vi "Volume Matcher.vi"() -> ()   [LabVIEW 2024, in "CLZ_to_ComicVine.lvlib"]
uses:
  CLZ_to_ComicVine.lvlib
  Volumes/CV Comics.lvclass
  CLZ Comics/CLZ Comics.lvclass
  <vilib>/Utility/miscctls.llb/LVRowAndColumnUnsignedTypeDef.ctl
  <vilib>/addons/_JKI Toolkits/State Machine/_JKI_lib_State_Machine.llb/Select State(s)_err__jki_lib_state_machine.vi
  <vilib>/addons/_JKI Toolkits/State Machine/_JKI_lib_State_Machine.llb/Periodic Trigger__ogtk__JKI-SM__jki_lib_state_machine.vi
panel:
  in  "Matched Volumes":i32(listbox)
  in  "CLZ Issues":i32(listbox)
  in  "regex":string
  in  "Sort Type":enum16{"Fuzzy", "Regex"}(ring)
  in  "refresh":bool
  in  "compare threshold":dbl=0.5 min=0.0 max=1.0 step=0.1
  out "progress":i32(slide) caption="1582 of 1626" scale=0.0..1626.0
  in  "Remove Set":bool
  in  "Apply Set":bool
  in  "CV Volumes":i32(listbox)
  in  "CLZ Volumes":i32(listbox)
  in  "Exit":bool
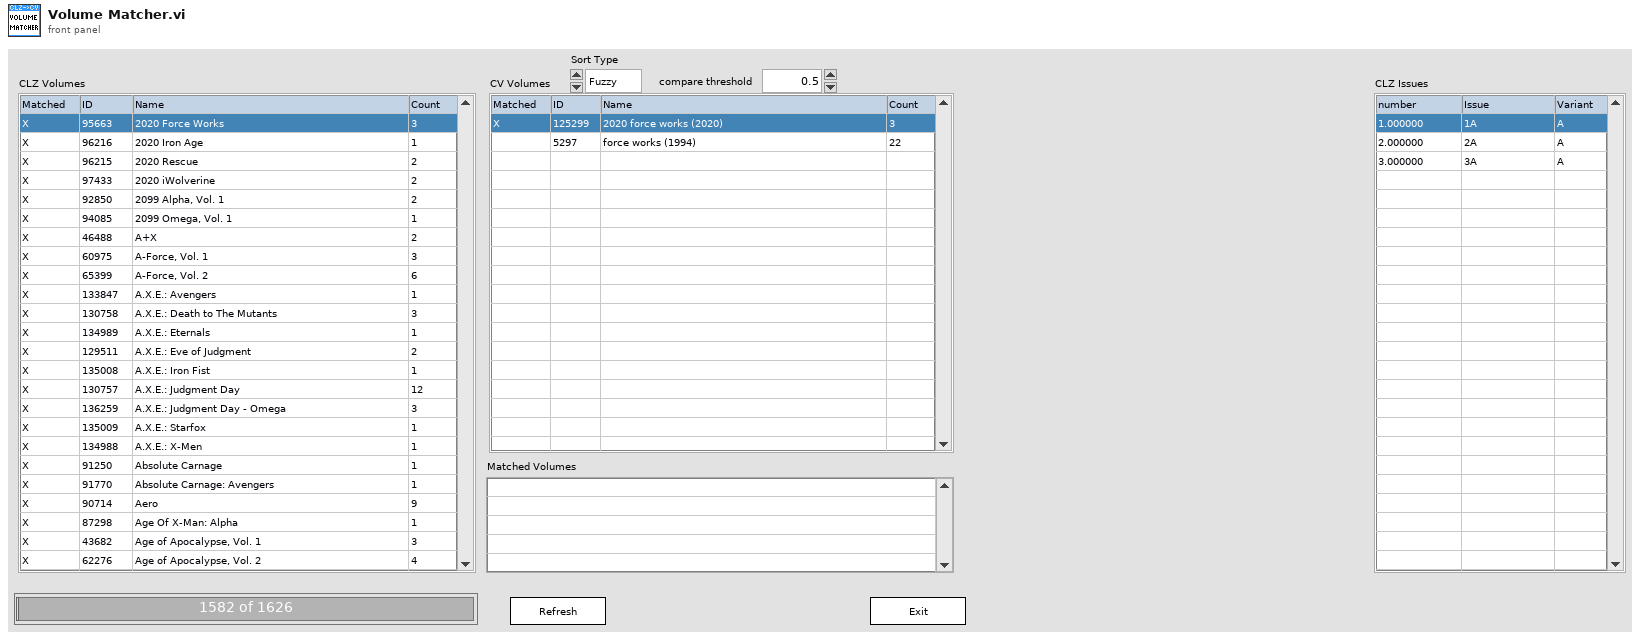
[diagram p1: front panel]
types:
  T1 = enum32{"Invalid", "Standard", "Closed", "Hidden", "Minimized", "Maximized"}
  T2 = enum32{"invalid app kind", "Development System", "Run Time System", "Student Edition", "Embedded LabVIEW", "Evaluation", "Custom"}
  T3 = cluster{"Core":cluster{"Current VI Reference":refnum<vi>, "Close Panel on Exit?":bool}, "CLZ report path":path, "CV binary folder":path, "matched set":set{cluster{"CLZ ID":i32, "CV ID":i32}}, "CLZ Comics":refnum<class "CLZ Comics.lvclass">, "CV volumes":refnum<class "CV Comics.lvclass">}
  T4 = cluster{"Current VI Reference":refnum<vi>, "Close Panel on Exit?":bool}
  T5 = typedef "LVRowAndColumnUnsignedTypeDef.ctl" = cluster{"Row":u32, "Column":u32}
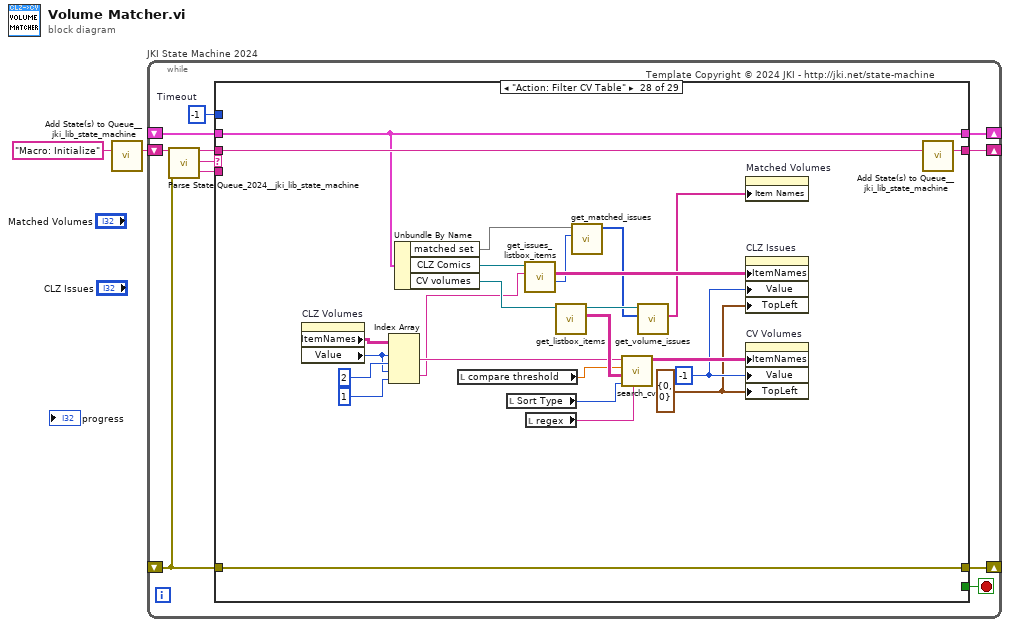
[diagram p0: block diagram]
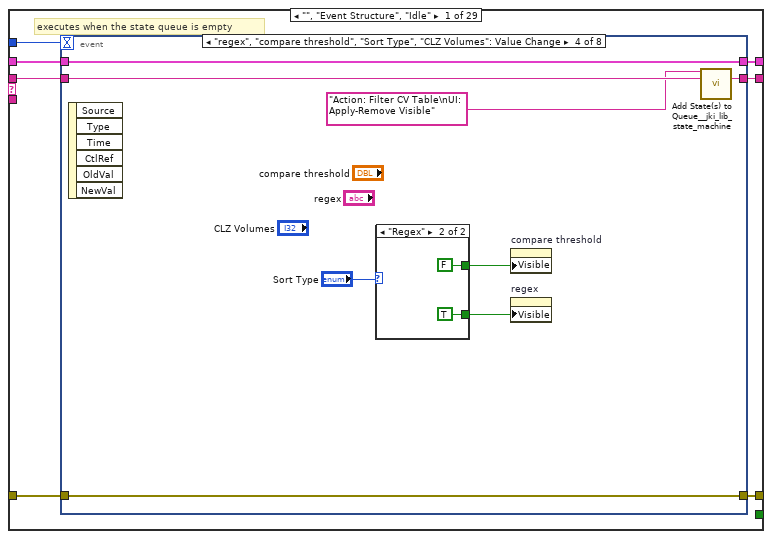
[diagram p2: hidden frame]
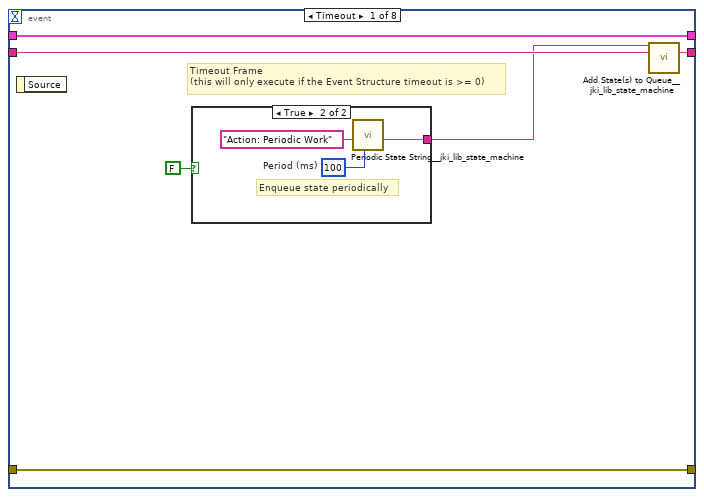
[diagram p3: hidden frame]
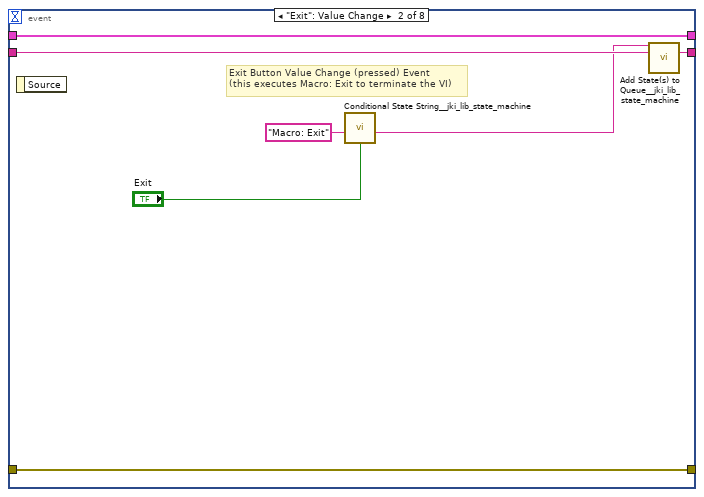
[diagram p5: hidden frame]
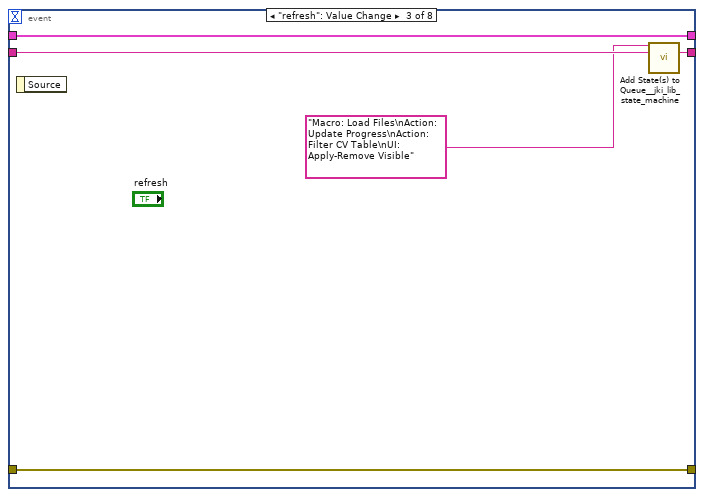
[diagram p6: hidden frame]
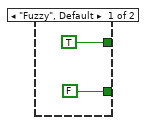
[diagram p7: hidden frame]
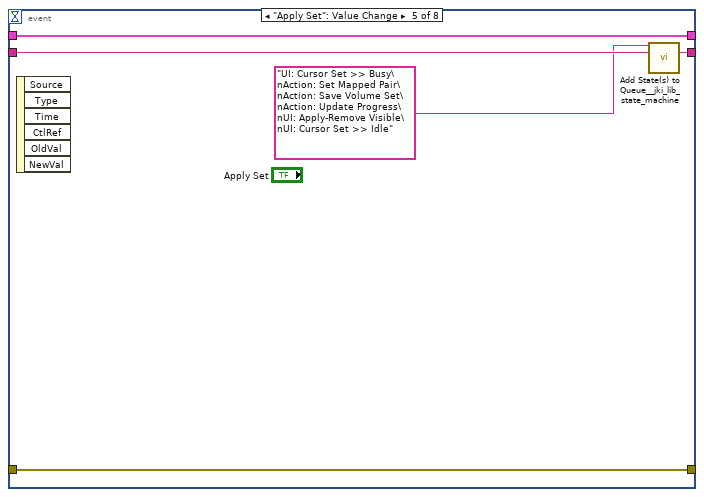
[diagram p8: hidden frame]
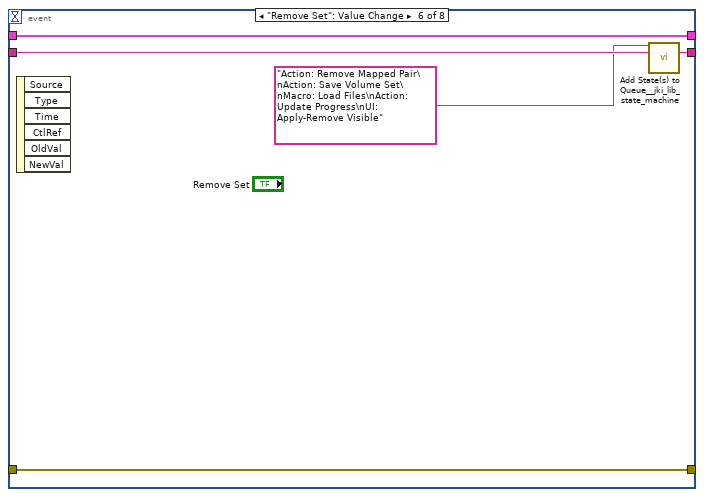
[diagram p9: hidden frame]
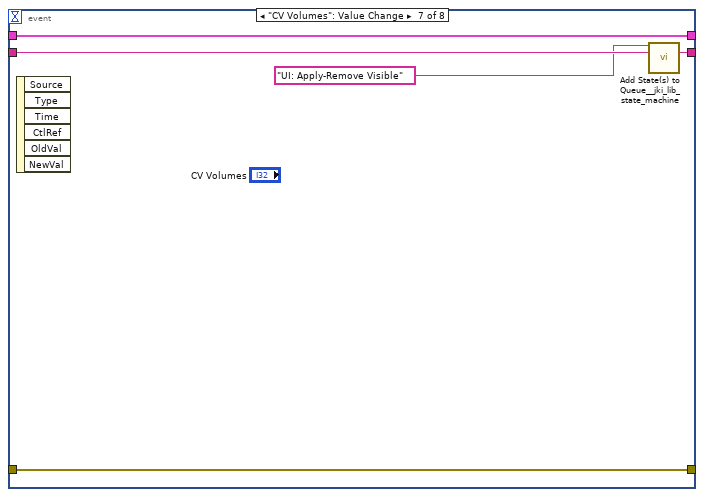
[diagram p10: hidden frame]
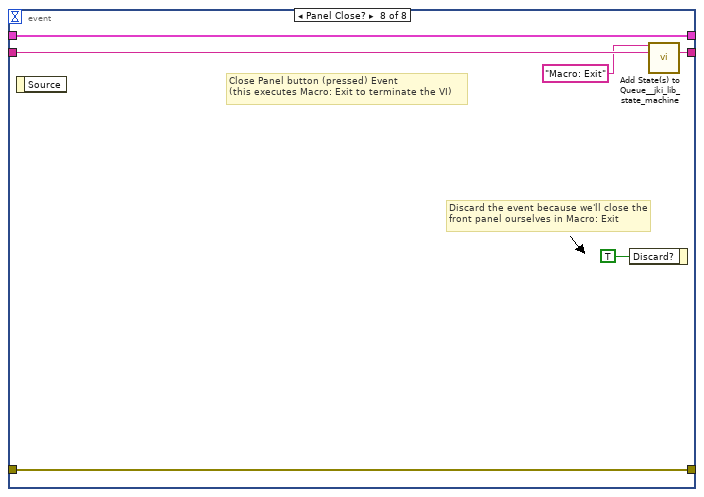
[diagram p11: hidden frame]
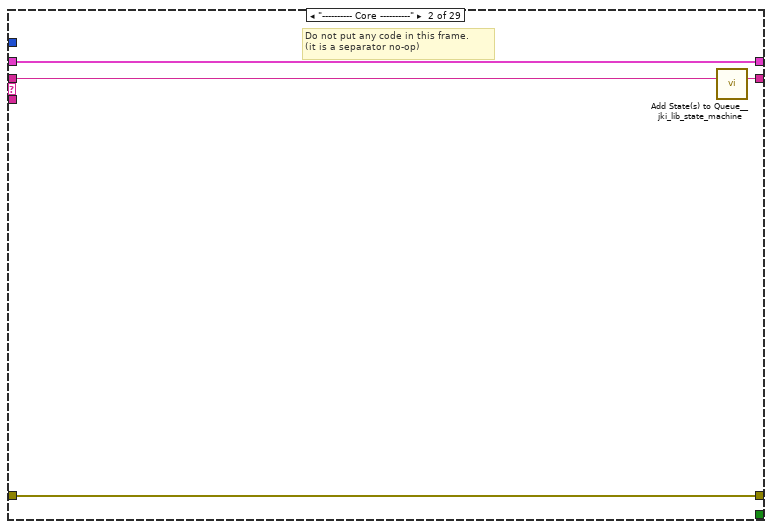
[diagram p12: hidden frame]
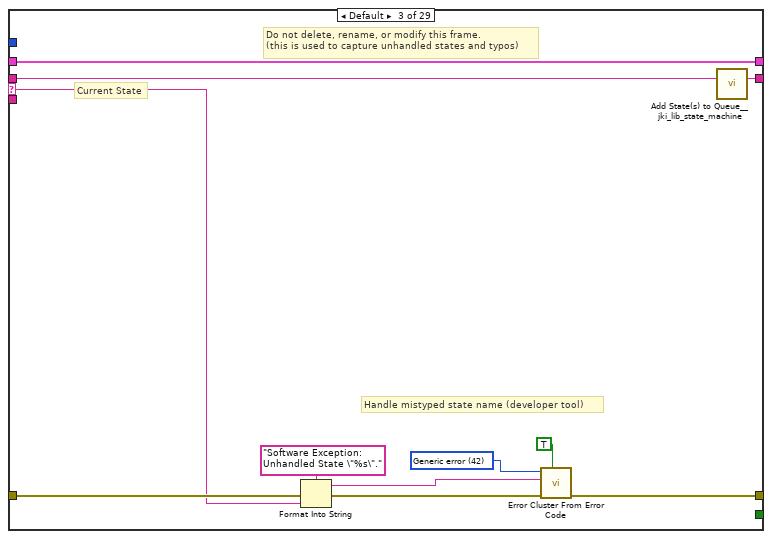
[diagram p13: hidden frame]
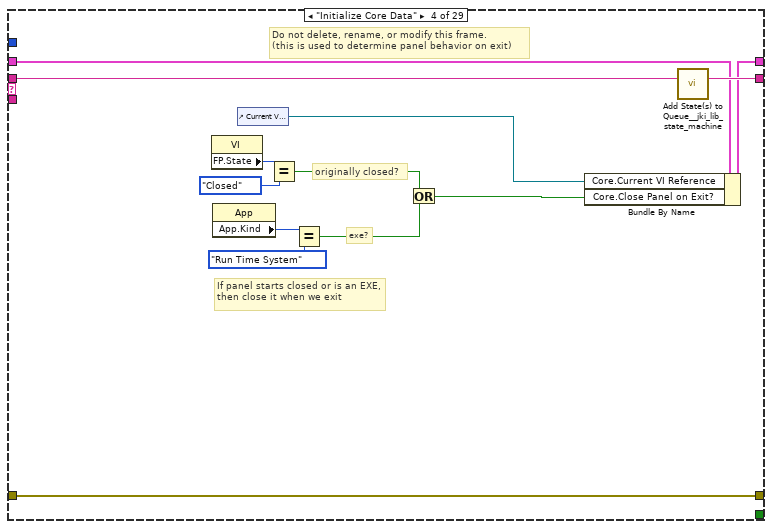
[diagram p14: hidden frame]
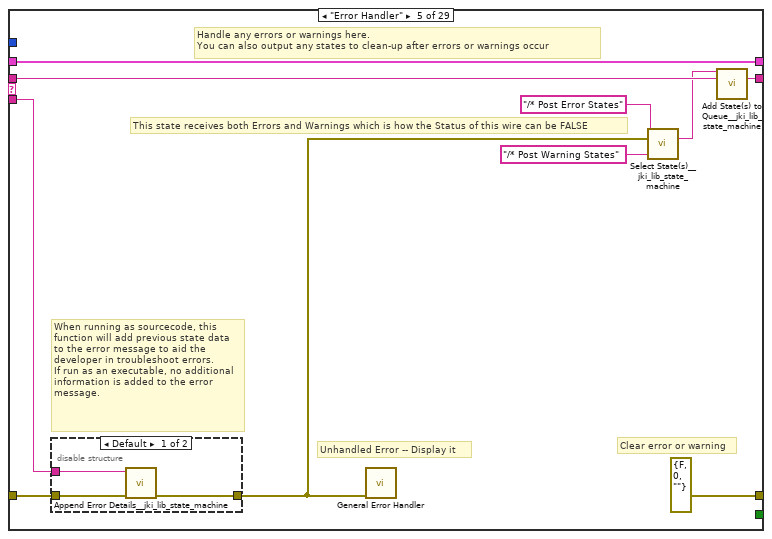
[diagram p15: hidden frame]
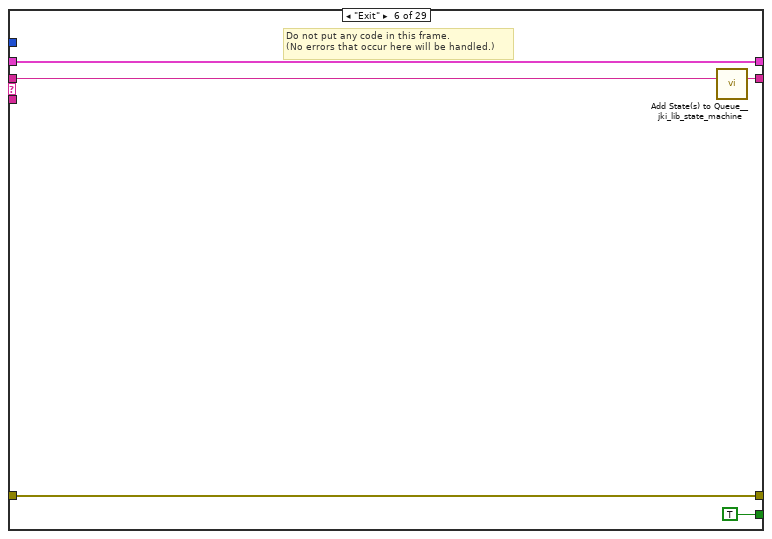
[diagram p17: hidden frame]
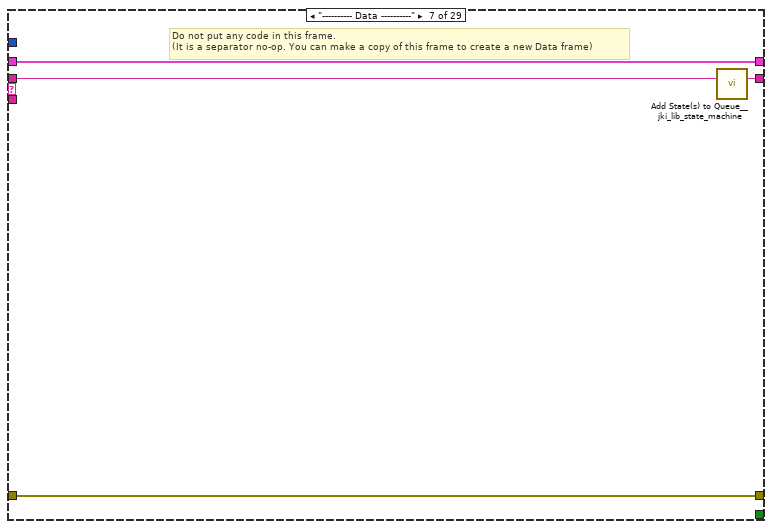
[diagram p18: hidden frame]
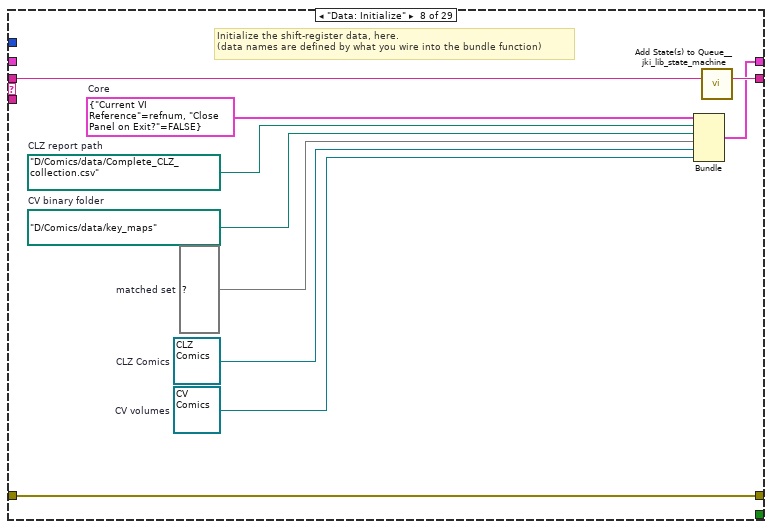
[diagram p19: hidden frame]
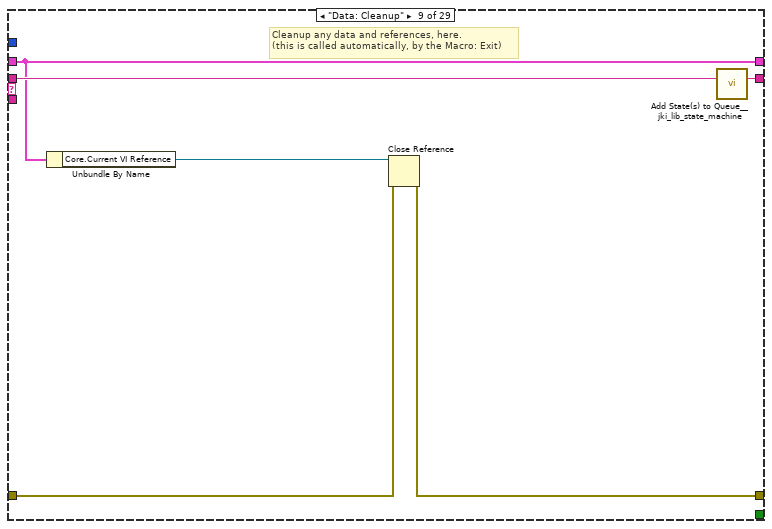
[diagram p20: hidden frame]
diagram:
  n1 = call <vilib>:"Add State(s) to Queue__jki_lib_state_machine.vi"("State(s) in (\"\")"="Macro: Initialize") -> ("States Out"=w2:string)  [unwired: 14 in]
  n2 = while "JKI State Machine 2024" {
    shift-right: [w6] -> _
    shift-left: _ -> [w5]
    shift-right: [w9] -> _
    shift-left: _ -> [w3]
    shift-right: [w8] -> _
    shift-left: w2 -> [w10]
    stop <- w7 stop-if-true
    w4 = -1  # Timeout
    # "Template Copyright © 2024 JKI - http://jki.net/state-machine"
    n3 = call <vilib>:"Parse State Queue_2024__jki_lib_state_machine.vi"("State Queue"=w10, "Error In (no error)"=w3) -> ("Remaining States"=w12:string, "Current State"=w13:string, "Arguments"=w11:string)  [unwired: 11 in]
    n4 = case shown="\"Action: Filter CV Table\"" w13 {
      selector: w13 -> [_ _ w79 _ _ _ _ _ _ _ _ _ _ _ _ _ _ _ _ _ _ _ _ _ _ _ _ _ _]
      tunnel: w12 -> [w20 w78 w83 w102 w112 w121 w125 w135 w141 w145 w167 w195 w201 w207 w218 w287 w292 w297 w306 w310 w317 w343 w365 w376 w386 w394 w403 w428 w438]
      tunnel: w11 -> [_ _ _ _ w107 _ _ _ _ _ _ _ _ w202 w212 _ _ _ _ _ _ _ _ _ _ _ _ _ _]
      tunnel: w5 -> [w18 w75 w81 w95 w109 w119 w122 _ w136 w142 w158 w193 w199 w205 w214 w284 w289 w294 w304 w307 w315 w327 w362 w374 w384 w392 w401 w423 w436]
      tunnel: [w17 w76 w85 w99 errorcluster {"status"=FALSE, "code"=0, "source"=""} ("error out") w118 w123 w132 w137 w143 w165 w192 w198 w203 w215 w285 w290 w295 w301 w308 w311 w341 w363 w370 w377 w387 w397 w426 w433] -> w9
      tunnel: w3 -> [w14 w76 w84 w99 w108 w118 w123 w132 w138 w143 w165 w192 w198 w204 w216 w285 w290 w295 w301 w308 w312 w341 w363 w373 w378 w388 w398 w426 w435]
      tunnel: [w19 w77 w82 w101 w111 w120 w124 w134 w140 w144 w166 w194 w200 w206 w217 w286 w291 w296 w305 w309 w316 w342 w364 w375 w385 w393 w402 w427 w437] -> w8
      tunnel: [_ _ _ _ _ TRUE _ _ _ _ _ _ _ _ _ _ _ _ _ _ _ _ _ _ _ _ _ _ _] -> w7
      tunnel: [w16 w75 w81 w100 w109 w119 w122 w133 w136 w142 w158 w193 w199 w205 w214 w284 w289 w294 w304 w307 w315 w326 w361 w374 w383 w391 w401 w423 w434] -> w6
      tunnel: w4 -> [w15 _ _ _ _ _ _ _ _ _ _ _ _ _ _ _ _ _ _ _ _ _ _ _ _ _ _ _ _]
      frame "", "Event Structure", "Idle" {
        # "executes when the state queue is empty"
        n5 = event shown="[3] \"regex\", \"compare threshold\", \"Sort Type\", \"CLZ Volumes\": Value Change" {
          selector: _ -> [_ _ _ _ _ _ _ _]
          dyn-events: _ -> [_ _ _ _ _ _ _ _]
          timeout: w15 -> [_ _ _ _ _ _ _ _]
          tunnel: w20 -> [w26 w36 w41 w49 w58 w63 w68 w74]
          tunnel: [w25 w35 w40 w48 w57 w62 w67 w73] -> w19
          tunnel: w18 -> [w23 w33 w38 w46 w55 w60 w65 w71]
          tunnel: [w24 w34 w39 w47 w56 w61 w66 w72] -> w17
          tunnel: w14 -> [w24 w34 w39 w47 w56 w61 w66 w72]
          tunnel: [w23 w33 w38 w46 w55 w60 w65 w71] -> w16
          event Timeout {
            # "Timeout Frame\n(this will only execute if the Event Structure timeout is >= 0)"
            n6 = event-data() -> ()  [unwired: 1 in, 1 out]
            n7 = case shown="True" FALSE {
              tunnel: [_ w29] -> w22
              frame False {
              }
              frame True {
                w27 = u32 100  # Period (ms)
                # "Enqueue state periodically"
                n8 = call <vilib>:"Periodic State String__jki_lib_state_machine.vi"("Period (ms)"=w27, "State"="Action: Periodic Work") -> ("State Out"=w29:string)  [unwired: 9 in]
              }
            }
            n9 = call <vilib>:"Add State(s) to Queue__jki_lib_state_machine.vi"("State(s) in Front (\"\")"=w22, "State(s) in (\"\")"=w26) -> ("States Out"=w25:string)  [unwired: 13 in]
          }
          event "Exit": Value Change {
            # "Exit Button Value Change (pressed) Event\n(this executes Macro: Exit to terminate the VI)"
            n10 = event-data() -> ()  [unwired: 1 in, 1 out]
            n11 = call <vilib>:"Conditional State String__jki_lib_state_machine.vi"("Do State(s)?"="Exit", "State"="Macro: Exit") -> ("State Out"=w30:string)  [unwired: 7 in]
            n12 = call <vilib>:"Add State(s) to Queue__jki_lib_state_machine.vi"("State(s) in Front (\"\")"=w30, "State(s) in (\"\")"=w36) -> ("States Out"=w35:string)  [unwired: 13 in]
          }
          event "refresh": Value Change {
            n13 = event-data() -> ()  [unwired: 1 in, 1 out]
            n14 = call <vilib>:"Add State(s) to Queue__jki_lib_state_machine.vi"("State(s) in Front (\"\")"="Macro: Load Files\nAction: Update Progress\nAction: Filter CV Table\nUI: Apply-Remove Visible" ("State(s) in Front (\"\")"), "State(s) in (\"\")"=w41) -> ("States Out"=w40:string)  [unwired: 13 in]
          }
          event "regex", "compare threshold", "Sort Type", "CLZ Volumes": Value Change {
            n15 = event-data() -> ()  [unwired: 1 in, 6 out]
            n16 = case shown="\"Regex\"" "Sort Type" {
              tunnel: [TRUE FALSE] -> w44
              tunnel: [FALSE TRUE] -> w43
              frame "Fuzzy", Default {
              }
              frame "Regex" {
              }
            }
            n17 = property on="compare threshold" class="DigNum (strict)"("Visible"=w44) -> ()  [unwired: 2 in, 2 out]
            n18 = property on="regex" class="Str"("Visible"=w43) -> ()  [unwired: 2 in, 2 out]
            n19 = call <vilib>:"Add State(s) to Queue__jki_lib_state_machine.vi"("State(s) in Front (\"\")"="Action: Filter CV Table\nUI: Apply-Remove Visible", "State(s) in (\"\")"=w49) -> ("States Out"=w48:string)  [unwired: 13 in]
          }
          event "Apply Set": Value Change {
            n20 = event-data() -> ()  [unwired: 1 in, 6 out]
            n21 = call <vilib>:"Add State(s) to Queue__jki_lib_state_machine.vi"("State(s) in Front (\"\")"="UI: Cursor Set >> Busy\nAction: Set Mapped Pair\nAction: Save Volume Set\nAction: Update Progress\nUI: Apply-Remove Visible\nUI: Cursor Set >> Idle", "State(s) in (\"\")"=w58) -> ("States Out"=w57:string)  [unwired: 13 in]
          }
          event "Remove Set": Value Change {
            n22 = event-data() -> ()  [unwired: 1 in, 6 out]
            n23 = call <vilib>:"Add State(s) to Queue__jki_lib_state_machine.vi"("State(s) in Front (\"\")"="Action: Remove Mapped Pair\nAction: Save Volume Set\nMacro: Load Files\nAction: Update Progress\nUI: Apply-Remove Visible", "State(s) in (\"\")"=w63) -> ("States Out"=w62:string)  [unwired: 13 in]
          }
          event "CV Volumes": Value Change {
            n24 = event-data() -> ()  [unwired: 1 in, 6 out]
            n25 = call <vilib>:"Add State(s) to Queue__jki_lib_state_machine.vi"("State(s) in Front (\"\")"="UI: Apply-Remove Visible", "State(s) in (\"\")"=w68) -> ("States Out"=w67:string)  [unwired: 13 in]
          }
          event Panel Close? {
            # "Discard the event because we'll close the front panel ourselves in Macro: Exit"
            # "Close Panel button (pressed) Event\n(this executes Macro: Exit to terminate the VI)"
            n26 = event-data() -> ()  [unwired: 1 in, 1 out]
            n27 = event-data("Discard?"=TRUE) -> ()  [unwired: 1 in, 1 out]
            n28 = call <vilib>:"Add State(s) to Queue__jki_lib_state_machine.vi"("State(s) in Front (\"\")"="Macro: Exit", "State(s) in (\"\")"=w74) -> ("States Out"=w73:string)  [unwired: 13 in]
          }
        }
      }
      frame "---------- Core ----------" {
        # "Do not put any code in this frame.\n(it is a separator no-op)"
        n29 = call <vilib>:"Add State(s) to Queue__jki_lib_state_machine.vi"("State(s) in (\"\")"=w78) -> ("States Out"=w77:string)  [unwired: 14 in]
      }
      frame Default {
        w88 = 42 items=["No error", "Argument error", "Memory is full", "Out of zone", "End of file", "File already open", "Generic file I/O error", "File not found", "File permission error", "Disk is full", "Duplicate path", "Too many files open", "System feature not enabled", "Resource file not found", "Cannot add resource", "Resource not found", "Image not found", "Image memory error", "Pen does not exist", "Config type invalid", "Config token not found", "Config parse error", "Config memory error", "Bad external code format", "Bad external code offset", "External code not present", "Null window", "Destroy window error", "Null menu", "Print aborted", "Bad print record", "Print driver error", "Windows error during printing", "Memory error during printing", "Print dialog error", "Generic print error", "Invalid device refnum", "Device not found", "Device parameter error", "Device unit error", "Cannot open device", "Device call aborted", "Generic error", "Cancelled by user", "Object ID too low", "Object ID too high", "Object not in heap", "Unknown heap", "Unknown object (invalid DefProc)", "Unknown object (DefProc not in table)", "Message out of range", "Invalid (null) method", "Unknown message", "Manager call not supported", "Bad address", "Network operation in progress", "Network operation timed out", "Connection is busy", "Network attribute not supported", "Network error", "Address in use", "System out of memory", "Connection aborted", "Connection refused", "Not connected", "Already connected", "Connection closed", "Initialization error (interapplication manager)", "Bad occurrence", "Wait on unbound occurrence handler", "Occurrence queue overflow", "Datalog type conflict", "Unused", "Unrecognized type (interapplication manager)", "Memory corrupt", "Failed to make temporary DLL", "Old CIN version", "Drag socket not found", "Failed to load drop-object", "Failed to register OLE object", "Failed to release OLE object", "Format specifier type mismatch", "Unknown format specifier", "Too few format specifiers", "Too many format specifiers", "Scan failed", "Newer CIN version", "Error converting to variant", "Runtime menu error", "Password tampered", "Variant attribute not found", "Incompatible variant data type", "Event data is not available", "Event Store is not present", "Occurrence is not found", "Event Queue is not created", "Event info is not available", "Refnum passed is NULL", "Error retrieving Class GUID", "Error retrieving CoClass GUID", "Error retrieving TypeLib GUID.", "Bad built application magic bytes.", "Specific driver is different from the specific driver associated with the Logical Name.", "There is no session opened to the class driver.", "Max Error", "MAX - Error with config objects", "MAX - Error loading configuration", "MAX - Group not supported"]
        # "Current State"
        # "Do not delete, rename, or modify this frame.\n(this is used to capture unhandled states and typos)"
        # "Handle mistyped state name (developer tool)"
        n30 = Format Into String(format string="Software Exception: Unhandled State \"%s\"." ("message"), error in=w84, w79) -> (resulting string=w87:string, error out=w86:errorcluster)  [unwired: 1 in]
        n31 = call <vilib>:"Error Cluster From Error Code.vi"("show call chain? (False)"=TRUE, "error in (no error)"=w86, "error message (\"\")"=w87, "error code (0)"=w88) -> ("error out"=w85:errorcluster)  [unwired: 5 in]
        n32 = call <vilib>:"Add State(s) to Queue__jki_lib_state_machine.vi"("State(s) in (\"\")"=w83) -> ("States Out"=w82:string)  [unwired: 14 in]
      }
      frame "Initialize Core Data" {
        # "Do not delete, rename, or modify this frame.\n(this is used to determine panel behavior on exit)"
        # "originally closed?"
        # "exe?"
        # "If panel starts closed or is an EXE, then close it when we exit"
        n33 = property class="VI"() -> ("FP.State"=w92:T1)  [unwired: 2 in, 2 out]
        n34 = property class="App"() -> ("App.Kind"=w98:T2)  [unwired: 2 in, 2 out]
        n35 = control-ref of="Current VI Reference"() -> (w93:refnum<vi>)
        n36 = Equal?(x=w92, y=T1."Closed" ("Front Panel Window:State")) -> (x = y?=w90:bool)
        n37 = Equal?(x=w98, y=T2."Run Time System" ("Application:Kind")) -> (x = y?=w96:bool)
        n38 = Or(x=w90, y=w96) -> (x .or. y?=w94:bool)
        n39 = Bundle By Name(cluster=w95, "Core.Current VI Reference"=w93, "Core.Close Panel on Exit?"=w94) -> (w100:T3)
        n40 = call <vilib>:"Add State(s) to Queue__jki_lib_state_machine.vi"("State(s) in (\"\")"=w102) -> ("States Out"=w101:string)  [unwired: 14 in]
      }
      frame "Error Handler" {
        # "When running as sourcecode, this function will add previous state data to the error message to aid the developer in troubleshoot errors.\nIf run as an executable, no additional information is added to the error message."
        # "This state receives both Errors and Warnings which is how the Status of this wire can be FALSE"
        # "Unhandled Error -- Display it"
        # "Handle any errors or warnings here.\nYou can also output any states to clean-up after errors or warnings occur"
        # "Clear error or warning"
        n41 = disable-structure shown="Default" {
          disable-tunnel: w108 -> [w115 w116]
          disable-tunnel: w107 -> [w114 _]
          disable-tunnel: [w113 w116] -> w106
          frame condition #0 (active) {
            n42 = call <vilib>:"Append Error Details__jki_lib_state_machine.vi"("error in (no error)"=w115, "Previous State and Argument(s)"=w114) -> ("error out"=w113:errorcluster)  [unwired: 9 in]
          }
          frame condition #1 {
          }
        }
        n43 = call <vilib>:"General Error Handler.vi"("error in (no error)"=w106) -> ()  [unwired: 10 in, 5 out]
        n44 = call-poly <vilib>:"Select State(s)__jki_lib_state_machine.vi"("State(s) if True (\"\")"="/* Post Error States", "Select"=w106, "State(s) if False (\"\")"="/* Post Warning States") -> ("States Out"=w104:string)  [unwired: 12 in]
        n45 = call <vilib>:"Add State(s) to Queue__jki_lib_state_machine.vi"("State(s) in Front (\"\")"=w104, "State(s) in (\"\")"=w112) -> ("States Out"=w111:string)  [unwired: 13 in]
      }
      frame "Exit" {
        # "Do not put any code in this frame.\n(No errors that occur here will be handled.)"
        n46 = call <vilib>:"Add State(s) to Queue__jki_lib_state_machine.vi"("State(s) in (\"\")"=w121) -> ("States Out"=w120:string)  [unwired: 14 in]
      }
      frame "---------- Data ----------" {
        # "Do not put any code in this frame.\n(It is a separator no-op. You can make a copy of this frame to create a new Data frame)"
        n47 = call <vilib>:"Add State(s) to Queue__jki_lib_state_machine.vi"("State(s) in (\"\")"=w125) -> ("States Out"=w124:string)  [unwired: 14 in]
      }
      frame "Data: Initialize" {
        w126 = refnum<class "CLZ Comics.lvclass"> refnum  # CLZ Comics
        w127 = refnum<class "CV Comics.lvclass"> refnum  # CV volumes
        w128 = set{cluster{"CLZ ID":i32, "CV ID":i32}} {}  # matched set
        w129 = path "D:/Comics/data/key_maps"  # CV binary folder
        w130 = path "D:/Comics/data/Complete_CLZ_collection.csv"  # CLZ report path
        w131 = T4 {"Current VI Reference"=refnum, "Close Panel on Exit?"=FALSE}  # Core
        # "Initialize the shift-register data, here.\n(data names are defined by what you wire into the bundle function)"
        n48 = Bundle("Core"=w131, "CLZ report path"=w130, "CV binary folder"=w129, "matched set"=w128, "CLZ Comics"=w126, "CV volumes"=w127) -> (w133:T3)  [unwired: 1 in]
        n49 = call <vilib>:"Add State(s) to Queue__jki_lib_state_machine.vi"("State(s) in (\"\")"=w135) -> ("States Out"=w134:string)  [unwired: 14 in]
      }
      frame "Data: Cleanup" {
        # "Cleanup any data and references, here.\n(this is called automatically, by the Macro: Exit)"
        n50 = Unbundle By Name(w136) -> ("Core.Current VI Reference"=w139:refnum<vi>)
        n51 = Close Reference(reference=w139, error in (no error)=w138) -> (error out=w137:errorcluster)
        n52 = call <vilib>:"Add State(s) to Queue__jki_lib_state_machine.vi"("State(s) in (\"\")"=w141) -> ("States Out"=w140:string)  [unwired: 14 in]
      }
      frame "---------- UI ----------" {
        # "Do not put any code in this frame.\n(It is a separator no-op. You can make a copy of this frame to create a new UI frame)"
        n53 = call <vilib>:"Add State(s) to Queue__jki_lib_state_machine.vi"("State(s) in (\"\")"=w145) -> ("States Out"=w144:string)  [unwired: 14 in]
      }
      frame "UI: Apply-Remove Visible" {
        n54 = property on="CLZ Volumes" class="MCListbox (strict)"() -> ("ItemNames"=w164:string[][], "Value"=w153:i32)  [unwired: 2 in, 2 out]
        n55 = property on="CV Volumes" class="MCListbox (strict)"() -> ("ItemNames"=w161:string[][], "Value"=w152:i32)  [unwired: 2 in, 2 out]
        n56 = Greater Or Equal To 0?(x=w153) -> (x >= 0?=w151:bool)
        n57 = Greater Or Equal To 0?(x=w152) -> (x >= 0?=w150:bool)
        n58 = And(x=w151, y=w150) -> (x .and. y?=w147:bool)
        n59 = Unbundle By Name(w158) -> ("matched set"=w157:set{cluster{"CLZ ID":i32, "CV ID":i32}})
        n60 = case shown="True" w147 {
          tunnel: w164 -> [_ w180]
          tunnel: [_ w178] -> w163
          tunnel: [_ w177] -> w162
          tunnel: w161 -> [_ w175]
          tunnel: [_ w170] -> w156
          tunnel: w153 -> [_ w169]
          tunnel: w152 -> [_ w168]
          frame False {
          }
          frame True {
            n61 = Index Array(array=w180, index (row) #1=w169, index (col) #1=0 ("disabled index (col)")) -> (element #1=w178:string, element #2=w174:string)  [unwired: 2 in]
            n62 = Index Array(array=w175, index (row) #1=w168, index (col) #1=0 ("disabled index (col)")) -> (element #1=w177:string, element #2=w173:string)  [unwired: 2 in]
            n63 = Decimal String To Number(string=w174) -> (number=w172:i32)  [unwired: 2 in, 1 out]
            n64 = Decimal String To Number(string=w173) -> (number=w171:i32)  [unwired: 2 in, 1 out]
            n65 = Bundle(w172, w171) -> (w170:cluster{i32, i32})  [unwired: 1 in]
          }
        }
        n66 = Element of Set?(10:w156, 11:w157) -> (3:w146:bool)
        n67 = Empty String/Path?(string/path=w163) -> (empty?=w159:bool)
        n68 = Empty String/Path?(string/path=w162) -> (empty?=w160:bool)
        n69 = Or(x=w159, y=w160) -> (x .or. y?=w148:bool)
        n70 = Not Or(1:w160, 2:w159) -> (0:w155:bool)
        n71 = Compound Arithmetic op=AND(w147, w155, w146) -> (w154:bool)
        n72 = Compound Arithmetic op=AND(invert w146, w147, w148) -> (w149:bool)
        n73 = property on="Apply Set" class="Bool (strict)"("Visible"=w149) -> ()  [unwired: 2 in, 2 out]
        n74 = property on="Remove Set" class="Bool (strict)"("Visible"=w154) -> ()  [unwired: 2 in, 2 out]
        n75 = call <vilib>:"Add State(s) to Queue__jki_lib_state_machine.vi"("State(s) in (\"\")"=w167) -> ("States Out"=w166:string)  [unwired: 14 in]
      }
      frame "UI: Initialize" {
        w181 = T5 {"Row"=0, "Column"=0} ("Top Left Visible Cell")
        w182 = string[][] []
        w190 = string[] ["Matched", "ID", "Name", "Count"] ("Row Header Strings[]")
        w191 = u32 4 ("Number of Columns")
        # "Initialize the User Interface, here.\n(this is called automatically, by the Macro: Initialize)"
        n76 = property on="CLZ Issues" class="MCListbox (strict)"("NumCols"=u32 3 ("Number of Columns"), "ColHdrString"=string[] ["number", "Issue", "Variant"], "ItemNames"=w182, "TopLeft"=w181) -> ()  [unwired: 2 in, 2 out]
        n77 = property on="CLZ Volumes" class="MCListbox (strict)"("NumCols"=w191, "ColHdrString"=w190, "ItemNames"=w182, "TopLeft"=w181) -> ()  [unwired: 2 in, 2 out]
        n78 = property on="CV Volumes" class="MCListbox (strict)"("NumCols"=w191, "ColHdrString"=w190, "ItemNames"=w182, "TopLeft"=w181) -> ()  [unwired: 2 in, 2 out]
        n79 = local write "Sort Type"(enum16{"Fuzzy", "Regex"}."Fuzzy" ("Sort Type")) -> ()
        n80 = property on="Apply Set" class="Bool (strict)"("Visible"=FALSE) -> ()  [unwired: 2 in, 2 out]
        n81 = property on="Remove Set" class="Bool (strict)"("Visible"=FALSE) -> ()  [unwired: 2 in, 2 out]
        n82 = property on="compare threshold" class="DigNum (strict)"("Visible"=TRUE) -> ()  [unwired: 2 in, 2 out]
        n83 = property on="regex" class="Str"("Visible"=FALSE) -> ()  [unwired: 2 in, 2 out]
        n84 = call <vilib>:"Add State(s) to Queue__jki_lib_state_machine.vi"("State(s) in (\"\")"=w195) -> ("States Out"=w194:string)  [unwired: 14 in]
      }
      frame "UI: Uninitialize" {
        # "Cleanup the User Interface, here.\n(this is called automatically, by the Macro: Exit)"
        n85 = property on="Apply Set" class="Bool (strict)"("Visible"=TRUE) -> ()  [unwired: 2 in, 2 out]
        n86 = property on="Remove Set" class="Bool (strict)"("Visible"=TRUE) -> ()  [unwired: 2 in, 2 out]
        n87 = call <vilib>:"Add State(s) to Queue__jki_lib_state_machine.vi"("State(s) in (\"\")"=w201) -> ("States Out"=w200:string)  [unwired: 14 in]
      }
      frame "UI: Cursor Set" {
        # "Argument"
        # "Set and Unset Cursor Busy.\n(Usage: \"UI: Cursor Set >> Busy|Idle\")"
        n88 = case shown="\"Idle\", Default" w202 {
          tunnel: w204 -> [w209 w211]
          tunnel: [w208 w210] -> w203
          frame "Idle", Default {
            n89 = call <vilib>:"Unset Busy.vi"("error in (no error)"=w209) -> ("error out"=w208:errorcluster)  [unwired: 10 in]
          }
          frame "Busy" {
            n90 = call <vilib>:"Set Busy.vi"("error in (no error)"=w211) -> ("error out"=w210:errorcluster)  [unwired: 9 in, 1 out]
          }
        }
        n91 = call <vilib>:"Add State(s) to Queue__jki_lib_state_machine.vi"("State(s) in (\"\")"=w207) -> ("States Out"=w206:string)  [unwired: 14 in]
      }
      frame "UI: Front Panel State" {
        # "Argument"
        # "Set Front Panel Open or Closed\n(Usage: \"UI: Front Panel State >> Open|Close\")"
        n92 = Unbundle By Name(w214) -> ("Core.Current VI Reference"=w213:refnum<vi>)
        n93 = case shown="\"Minimize\", \"Minimized\"" w212 {
          tunnel: w216 -> [w224 w239 w250 w263 w276]
          tunnel: [w226 w240 w252 w265 w278] -> w215
          tunnel: w213 -> [w225 w237 w251 w264 w277]
          frame "Open", "Standard", Default {
            w219 = T1."Standard" ("State")
            n94 = property class="VI"(reference=w225, error in=w224) -> (reference out=w222:refnum<vi>, error out=w223:errorcluster, "FP.State"=w221:T1)
            n95 = Not Equal?(x=w221, y=w219) -> (x != y?=w220:bool)
            n96 = case shown="True" w220 {
              tunnel: [w230 w232] -> w226
              tunnel: w223 -> [w229 w232]
              tunnel: w222 -> [w228 _]
              tunnel: w219 -> [w227 _]
              frame True {
                n97 = invoke class="VI" method="FP.Open"(reference=w228, error in=w229, "Activate"=TRUE, "State"=w227) -> (error out=w230:errorcluster)  [unwired: 1 in, 4 out]
              }
              frame False {
              }
            }
          }
          frame "Close", "Closed" {
            n98 = property class="VI"(reference=w237, error in=w239) -> (reference out=w236:refnum<vi>, error out=w238:errorcluster, "FP.State"=w234:T1)
            n99 = Not Equal?(x=w234, y=T1."Closed" ("Front Panel Window:State")) -> (x != y?=w233:bool)
            n100 = case shown="True" w233 {
              tunnel: [w241 w244] -> w240
              tunnel: w238 -> [w241 w243]
              tunnel: w236 -> [_ w242]
              frame False {
              }
              frame True {
                n101 = invoke class="VI" method="FP.Close"(reference=w242, error in=w243) -> (error out=w244:errorcluster)  [unwired: 1 in, 2 out]
              }
            }
          }
          frame "Hidden", "Hide" {
            w245 = T1."Hidden" ("State")
            n102 = property class="VI"(reference=w251, error in=w250) -> (reference out=w248:refnum<vi>, error out=w249:errorcluster, "FP.State"=w247:T1)
            n103 = Not Equal?(x=w247, y=w245) -> (x != y?=w246:bool)
            n104 = case shown="True" w246 {
              tunnel: [w256 w257] -> w252
              tunnel: w249 -> [w255 w257]
              tunnel: w248 -> [w254 _]
              tunnel: w245 -> [w253 _]
              frame True {
                n105 = invoke class="VI" method="FP.Open"(reference=w254, error in=w255, "State"=w253) -> (error out=w256:errorcluster)  [unwired: 2 in, 4 out]
              }
              frame False {
              }
            }
          }
          frame "Minimize", "Minimized" {
            w258 = T1."Minimized" ("State")
            n106 = property class="VI"(reference=w264, error in=w263) -> (reference out=w261:refnum<vi>, error out=w262:errorcluster, "FP.State"=w260:T1)
            n107 = Not Equal?(x=w260, y=w258) -> (x != y?=w259:bool)
            n108 = case shown="True" w259 {
              tunnel: [w269 w270] -> w265
              tunnel: w262 -> [w268 w270]
              tunnel: w261 -> [w267 _]
              tunnel: w258 -> [w266 _]
              frame True {
                n109 = invoke class="VI" method="FP.Open"(reference=w267, error in=w268, "State"=w266) -> (error out=w269:errorcluster)  [unwired: 2 in, 4 out]
              }
              frame False {
              }
            }
          }
          frame "Maximize", "Maximized" {
            w271 = T1."Maximized" ("State")
            n110 = property class="VI"(reference=w277, error in=w276) -> (reference out=w274:refnum<vi>, error out=w275:errorcluster, "FP.State"=w273:T1)
            n111 = Not Equal?(x=w273, y=w271) -> (x != y?=w272:bool)
            n112 = case shown="True" w272 {
              tunnel: [w282 w283] -> w278
              tunnel: w275 -> [w281 w283]
              tunnel: w274 -> [w280 _]
              tunnel: w271 -> [w279 _]
              frame True {
                n113 = invoke class="VI" method="FP.Open"(reference=w280, error in=w281, "State"=w279) -> (error out=w282:errorcluster)  [unwired: 2 in, 4 out]
              }
              frame False {
              }
            }
          }
        }
        n114 = call <vilib>:"Add State(s) to Queue__jki_lib_state_machine.vi"("State(s) in (\"\")"=w218) -> ("States Out"=w217:string)  [unwired: 14 in]
      }
      frame "---------- Macro ----------" {
        # "Do not put any code in this frame.\n(It is a separator no-op. You can make a copy of this frame to create a new Macro frame)"
        n115 = call <vilib>:"Add State(s) to Queue__jki_lib_state_machine.vi"("State(s) in (\"\")"=w287) -> ("States Out"=w286:string)  [unwired: 14 in]
      }
      frame "Macro: Initialize" {
        w288 = "Data: Initialize\nInitialize Core Data\nUI: Initialize\nUI: Front Panel State >> Open\nMacro: Load Files\nAction: Update Progress"  # Data: Initialize Initialize Core Data UI: Initialize UI: Front Panel State >> Open Macro: Load Files Action: Update Progress
        # "Initialization Macro\n(This is called once, when the VI starts)"
        n116 = call <vilib>:"Add State(s) to Queue__jki_lib_state_machine.vi"("State(s) in Front (\"\")"=w288, "State(s) in (\"\")"=w292) -> ("States Out"=w291:string)  [unwired: 13 in]
      }
      frame "Macro: Load Files" {
        n117 = call <vilib>:"Add State(s) to Queue__jki_lib_state_machine.vi"("State(s) in Front (\"\")"="UI: Cursor Set >> Busy\nAction: Load Volume Set\nAction: Load CLZ Report\nAction: Load CV Binary\nAction: Populate Tables\nUI: Cursor Set >> Idle", "State(s) in (\"\")"=w297) -> ("States Out"=w296:string)  [unwired: 13 in]
      }
      frame "Macro: Exit" {
        # "Exit Macro\n(This is called once, when the VI exits)"
        n118 = Unbundle By Name(w304) -> ("Core.Close Panel on Exit?"=w299:bool)
        n119 = call <vilib>:"Conditional State String__jki_lib_state_machine.vi"("Do State(s)?"=w299, "State"="UI: Front Panel State >> Close") -> ("State Out"=w298:string)  [unwired: 7 in]
        n120 = call <vilib>:"Add State(s) to Queue__jki_lib_state_machine.vi"("State(s) in (\"\")"=w298, "State(s) at Back (\"\")"="UI: Uninitialize\nData: Cleanup\nExit") -> ("States Out"=w302:string)  [unwired: 13 in]
        n121 = call <vilib>:"Add State(s) to Queue__jki_lib_state_machine.vi"("State(s) in Front (\"\")"=w302, "State(s) in (\"\")"=w306) -> ("States Out"=w305:string)  [unwired: 13 in]
      }
      frame "---------- Action ----------" {
        n122 = call <vilib>:"Add State(s) to Queue__jki_lib_state_machine.vi"("State(s) in (\"\")"=w310) -> ("States Out"=w309:string)  [unwired: 14 in]
      }
      frame "Action: Update Progress" {
        n123 = Unbundle By Name(w315) -> ("CLZ Comics"=w314:refnum<class "CLZ Comics.lvclass">)
        n124 = control-ref of="progress"() -> (w313:refnum<vi>)
        n125 = call "update_progress_bar.vi"("error in (no error)"=w312, "progress ref"=w313, "Volumes in"=w314) -> ("error out"=w311:errorcluster)  [unwired: 7 in, 1 out]
        n126 = call <vilib>:"Add State(s) to Queue__jki_lib_state_machine.vi"("State(s) in (\"\")"=w317) -> ("States Out"=w316:string)  [unwired: 14 in]
      }
      frame "Action: Set Mapped Pair" {
        n127 = property on="CLZ Volumes" class="MCListbox (strict)"() -> ("ItemNames"=w340:string[][], "Value"=w338:i32)  [unwired: 2 in, 2 out]
        n128 = property on="CV Volumes" class="MCListbox (strict)"() -> ("ItemNames"=w331:string[][], "Value"=w333:i32)  [unwired: 2 in, 2 out]
        n129 = in-place {
          in-place-border: [w346] -> w330
          n130 = in-place-array #1(w340, w338, 0, w338, 1) -> (w346:string)  [unwired: 1 out]
          n131 = in-place-array #1("X" ("element"), w346) -> (w336:string[][])  [unwired: 4 out]
        }
        n132 = in-place {
          in-place-border: [w344] -> w329
          n133 = in-place-array #2(w331, w333, 0, w333, 1) -> (w344:string)  [unwired: 1 out]
          n134 = in-place-array #2("X" ("element"), w344) -> (w335:string[][])  [unwired: 4 out]
        }
        n135 = property on="CLZ Volumes" class="MCListbox (strict)"("ItemNames"=w336) -> ()  [unwired: 2 in, 2 out]
        n136 = property on="CV Volumes" class="MCListbox (strict)"("ItemNames"=w335) -> ()  [unwired: 2 in, 2 out]
        n137 = Decimal String To Number(string=w330) -> (number=w318:i32)  [unwired: 2 in, 1 out]
        n138 = Decimal String To Number(string=w329) -> (number=w323:i32)  [unwired: 2 in, 1 out]
        n139 = Unbundle By Name(w327) -> ("CLZ Comics"=w320:refnum<class "CLZ Comics.lvclass">, "CV volumes"=w328:refnum<class "CV Comics.lvclass">, "matched set"=w324:set{cluster{"CLZ ID":i32, "CV ID":i32}})
        n140 = Bundle(w318, w323) -> (w322:cluster{i32, i32})  [unwired: 1 in]
        n141 = call "set_id_mapped.vi"("ID"=w318, "Volumes in"=w320) -> ("Volumes out"=w319:refnum<class "CLZ Comics.lvclass">)  [unwired: 9 in]
        n142 = call "set_id_mapped.vi"("ID"=w323, "Volumes in"=w328) -> ("Volumes out"=w325:refnum<class "CV Comics.lvclass">)  [unwired: 9 in]
        n143 = Insert Into Set(10:w322, 11:w324) -> (3:w321:set{cluster{"CLZ ID":i32, "CV ID":i32}})  [unwired: 1 out]
        n144 = Bundle By Name(cluster=w327, "CLZ Comics"=w319, "CV volumes"=w325, "matched set"=w321) -> (w326:T3)
        n145 = call <vilib>:"Add State(s) to Queue__jki_lib_state_machine.vi"("State(s) in (\"\")"=w343) -> ("States Out"=w342:string)  [unwired: 14 in]
      }
      frame "Action: Remove Mapped Pair" {
        n146 = property on="CLZ Volumes" class="MCListbox (strict)"() -> ("ItemNames"=w355:string[][], "Value"=w354:i32)  [unwired: 2 in, 2 out]
        n147 = property on="CV Volumes" class="MCListbox (strict)"() -> ("ItemNames"=w350:string[][], "Value"=w349:i32)  [unwired: 2 in, 2 out]
        n148 = Index Array(array=w355, index (row)=w354, index (col)=1) -> (element=w352:string)
        n149 = Index Array(array=w350, index (row)=w349, index (col)=1) -> (element=w348:string)
        n150 = Unbundle By Name(w362) -> ("matched set"=w360:set{cluster{"CLZ ID":i32, "CV ID":i32}})
        n151 = Decimal String To Number(string=w352) -> (number=w359:i32)  [unwired: 2 in, 1 out]
        n152 = Decimal String To Number(string=w348) -> (number=w358:i32)  [unwired: 2 in, 1 out]
        n153 = Bundle(w359, w358) -> (w357:cluster{i32, i32})  [unwired: 1 in]
        n154 = Remove From Set(10:w357, 11:w360) -> (3:w356:set{cluster{"CLZ ID":i32, "CV ID":i32}})  [unwired: 1 out]
        n155 = Bundle By Name(cluster=w362, "matched set"=w356) -> (w361:T3)
        n156 = call <vilib>:"Add State(s) to Queue__jki_lib_state_machine.vi"("State(s) in (\"\")"=w365) -> ("States Out"=w364:string)  [unwired: 14 in]
      }
      frame "Action: Populate Tables" {
        n157 = Unbundle By Name(w374) -> ("CLZ Comics"=w367:refnum<class "CLZ Comics.lvclass">, "CV volumes"=w369:refnum<class "CV Comics.lvclass">)
        n158 = call "get_listbox_items.vi"("Volumes in"=w369) -> ("listbox items"=w368:string[][])  [unwired: 9 in, 1 out]
        n159 = call "get_volumes_listbox_items.vi"("Volumes in"=w367) -> ("listbox items"=w366:string[][])  [unwired: 9 in, 1 out]
        n160 = property on="CLZ Volumes" class="MCListbox (strict)"(error in=w373, "ItemNames"=w366) -> (error out=w372:errorcluster)  [unwired: 1 in, 1 out]
        n161 = property on="CV Volumes" class="MCListbox (strict)"("ItemNames"=w368) -> (error out=w371:errorcluster)  [unwired: 2 in, 1 out]
        n162 = Merge Errors(w372, w371) -> (w370:errorcluster)
        n163 = call <vilib>:"Add State(s) to Queue__jki_lib_state_machine.vi"("State(s) in (\"\")"=w376) -> ("States Out"=w375:string)  [unwired: 14 in]
      }
      frame "Action: Load CLZ Report" {
        n164 = Unbundle By Name(w384) -> ("matched set"=w380:set{cluster{"CLZ ID":i32, "CV ID":i32}}, "CLZ Comics"=w382:refnum<class "CLZ Comics.lvclass">, "CLZ report path"=w379:path)
        n165 = call "load_clz_data.vi"("matched set"=w380, "error in (no error)"=w378, "report path"=w379, "Volumes in"=w382) -> ("error out"=w377:errorcluster, "Volumes out"=w381:refnum<class "CLZ Comics.lvclass">)  [unwired: 6 in]
        n166 = Bundle By Name(cluster=w384, "CLZ Comics"=w381) -> (w383:T3)
        n167 = call <vilib>:"Add State(s) to Queue__jki_lib_state_machine.vi"("State(s) in (\"\")"=w386) -> ("States Out"=w385:string)  [unwired: 14 in]
      }
      frame "Action: Load Volume Set" {
        n168 = Unbundle By Name(w392) -> ("CV binary folder"=w390:path)
        n169 = call "read_volume_set.vi"("error in"=w388, "binary folder"=w390) -> ("error out"=w387:errorcluster, "matched set"=w389:set{cluster{"CLZ id":i32, "CV id":i32}})  [unwired: 8 in]
        n170 = Bundle By Name(cluster=w392, "matched set"=w389) -> (w391:T3)
        n171 = call <vilib>:"Add State(s) to Queue__jki_lib_state_machine.vi"("State(s) in (\"\")"=w394) -> ("States Out"=w393:string)  [unwired: 14 in]
      }
      frame "Action: Save Volume Set" {
        n172 = Unbundle By Name(w401) -> ("matched set"=w395:set{cluster{"CLZ ID":i32, "CV ID":i32}}, "CV binary folder"=w400:path)
        n173 = Build Path(base path=w400, name or relative path=path "volume_matched_set.bin") -> (appended path=w396:path)
        n174 = Write to Binary File(file (use dialog)=w396, data=w395, error in=w398) -> (error out=w397:errorcluster)  [unwired: 3 in, 2 out]
        n175 = call <vilib>:"Add State(s) to Queue__jki_lib_state_machine.vi"("State(s) in (\"\")"=w403) -> ("States Out"=w402:string)  [unwired: 14 in]
      }
      frame "Action: Filter CV Table" {
        w410 = T5 {"Row"=0, "Column"=0} ("Top Left Visible Cell")
        w411 = -1 ("CV Volumes")
        n176 = property on="CLZ Volumes" class="MCListbox (strict)"() -> ("ItemNames"=w425:string[][], "Value"=w415:i32)  [unwired: 2 in, 2 out]
        n177 = Index Array(array=w425, index (row) #1=w415, index (col) #1=2 ("disabled index (col)"), index (row) #2=w415, index (col) #2=1 ("disabled index (col)")) -> (element #1=w420:string, element #2=w409:string)
        n178 = Unbundle By Name(w423) -> ("matched set"=w408:set{cluster{"CLZ ID":i32, "CV ID":i32}}, "CLZ Comics"=w413:refnum<class "CLZ Comics.lvclass">, "CV volumes"=w422:refnum<class "CV Comics.lvclass">)
        n179 = local read "compare threshold"() -> (w418:dbl)
        n180 = local read "Sort Type"() -> (w417:enum16{"Fuzzy", "Regex"})
        n181 = call "get_issues_listbox_items.vi"("CLZ Vol ID"=w409, "CLZ Comics in"=w413) -> ("id"=w407:i32, "listbox contents"=w412:string[][])  [unwired: 7 in, 1 out]
        n182 = local read "regex"() -> (w416:string)
        n183 = call "get_listbox_items.vi"("Volumes in"=w422) -> ("listbox items"=w421:string[][], "Volumes out"=w406:refnum<class "CV Comics.lvclass">)  [unwired: 9 in]
        n184 = call "get_matched_issues.vi"("id"=w407, "matched set"=w408) -> ("matched cv ids"=w405:i32[])  [unwired: 9 in]
        n185 = call "search_cv.vi"("regex"=w416, "Sort Type"=w417, "Array in"=w421, "compare threshold"=w418, "search value"=w420) -> ("search results"=w419:string[][])  [unwired: 6 in]
        n186 = call "get_volume_issues.vi"("id"=w405, "CV Comics in"=w406) -> ("names"=w404:string[])  [unwired: 7 in, 2 out]
        n187 = property on="Matched Volumes" class="LstBox (strict)"("Item Names"=w404) -> ()  [unwired: 2 in, 2 out]
        n188 = property on="CLZ Issues" class="MCListbox (strict)"("ItemNames"=w412, "Value"=w411, "TopLeft"=w410) -> ()  [unwired: 2 in, 2 out]
        n189 = property on="CV Volumes" class="MCListbox (strict)"("ItemNames"=w419, "Value"=w411, "TopLeft"=w410) -> ()  [unwired: 2 in, 2 out]
        n190 = call <vilib>:"Add State(s) to Queue__jki_lib_state_machine.vi"("State(s) in (\"\")"=w428) -> ("States Out"=w427:string)  [unwired: 14 in]
      }
      frame "Action: Load CV Binary" {
        n191 = Unbundle By Name(w436) -> ("matched set"=w429:set{cluster{"CLZ ID":i32, "CV ID":i32}}, "CV binary folder"=w430:path, "CV volumes"=w432:refnum<class "CV Comics.lvclass">)
        n192 = call "load_cv_data.vi"("matched set"=w429, "error in (no error)"=w435, "binary folder"=w430, "Volumes in"=w432) -> ("error out"=w433:errorcluster, "Volumes out"=w431:refnum<class "CV Comics.lvclass">)  [unwired: 5 in, 1 out]
        n193 = Bundle By Name(cluster=w436, "CV volumes"=w431) -> (w434:T3)
        n194 = call <vilib>:"Add State(s) to Queue__jki_lib_state_machine.vi"("State(s) in (\"\")"=w438) -> ("States Out"=w437:string)  [unwired: 14 in]
      }
    }
  }
